vi "BackofDoor.vi"() -> ()   [LabVIEW 2017]
panel:
  in  "stop":bool
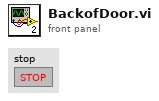
[diagram p1: front panel]
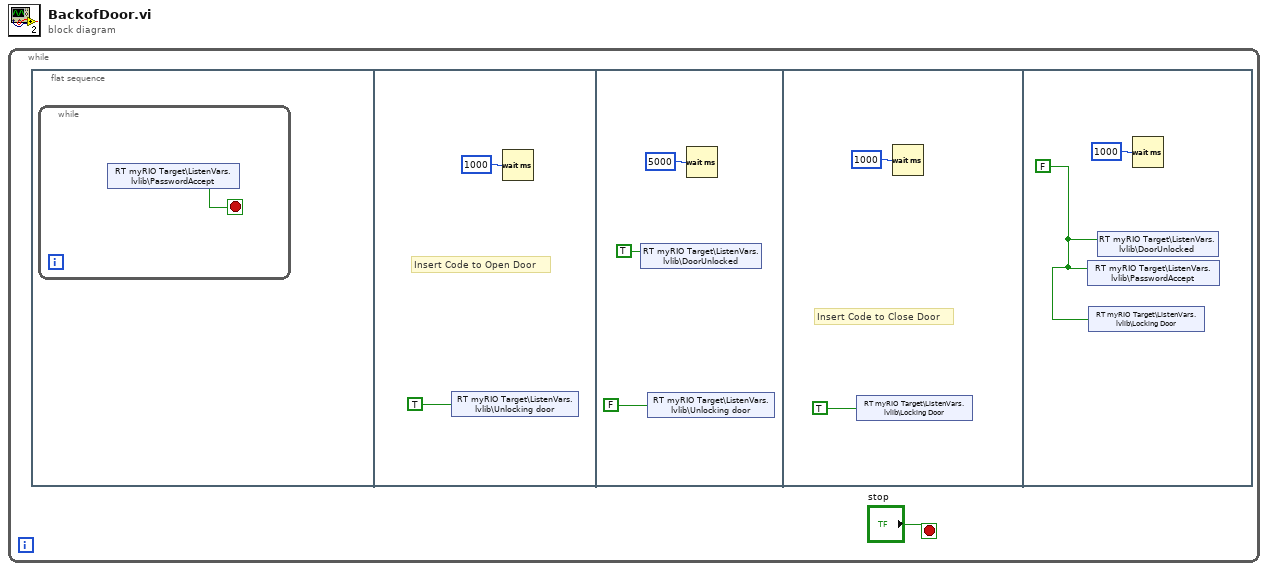
[diagram p0: block diagram]
diagram:
  n1 = while {
    stop <- "stop" stop-if-true
    n2 = flat-sequence {
      frame #0 {
        n3 = while {
          stop <- w2 stop-if-true
          n4 = shared-variable "RT myRIO Target\\ListenVars.lvlib\\PasswordAccept"() -> (w2:bool)  [unwired: 1 in, 1 out]
        }
      }
      frame #1 {
        # "Insert Code to Open Door"
        n5 = shared-variable "RT myRIO Target\\ListenVars.lvlib\\Unlocking door"(TRUE ("Unlocking Door")) -> ()  [unwired: 1 in, 1 out]
        n6 = Wait (ms)(milliseconds to wait=u32 1000) -> ()  [unwired: 1 out]
      }
      frame #2 {
        n7 = shared-variable "RT myRIO Target\\ListenVars.lvlib\\DoorUnlocked"(TRUE ("DoorUnlocked")) -> ()  [unwired: 1 in, 1 out]
        n8 = shared-variable "RT myRIO Target\\ListenVars.lvlib\\Unlocking door"(FALSE ("Unlocking Door")) -> ()  [unwired: 1 in, 1 out]
        n9 = Wait (ms)(milliseconds to wait=u32 5000) -> ()  [unwired: 1 out]
      }
      frame #3 {
        # "Insert Code to Close Door"
        n10 = shared-variable "RT myRIO Target\\ListenVars.lvlib\\Locking Door"(TRUE ("Unlocking Door")) -> ()  [unwired: 1 in, 1 out]
        n11 = Wait (ms)(milliseconds to wait=u32 1000) -> ()  [unwired: 1 out]
      }
      frame #4 {
        w11 = FALSE ("PasswordAccept")
        n12 = shared-variable "RT myRIO Target\\ListenVars.lvlib\\PasswordAccept"(w11) -> ()  [unwired: 1 in, 1 out]
        n13 = shared-variable "RT myRIO Target\\ListenVars.lvlib\\Locking Door"(w11) -> ()  [unwired: 1 in, 1 out]
        n14 = shared-variable "RT myRIO Target\\ListenVars.lvlib\\DoorUnlocked"(w11) -> ()  [unwired: 1 in, 1 out]
        n15 = Wait (ms)(milliseconds to wait=u32 1000) -> ()  [unwired: 1 out]
      }
    }
  }
